vi "process queue.vi"(6 "clear log?":bool, 10 "max log length (1000)":i32=1000, 11 "log queue":refnum<queue>) -> (2 "log items":string[](array[string]), 3 "# of items retrieved":i32)   [LabVIEW 2019, in "WebSocket Echo Server.lvlib"]
uses:
  WebSocket Echo Server.lvlib
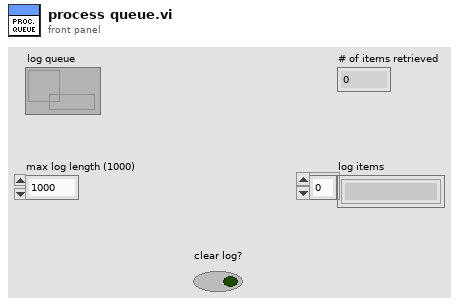
[diagram p1: front panel]
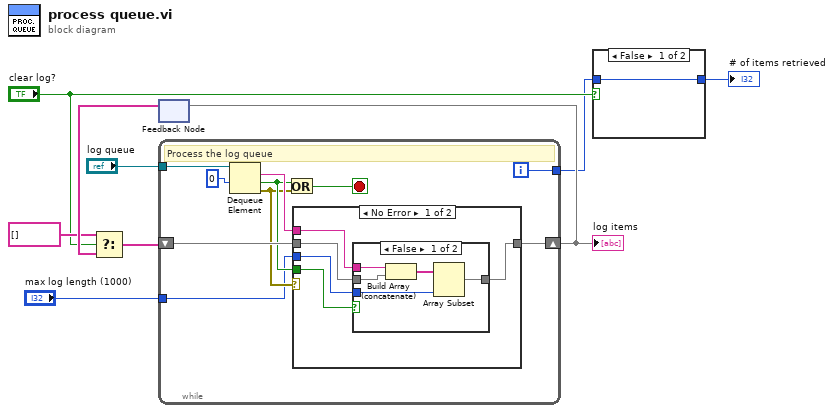
[diagram p0: block diagram]
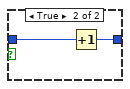
[diagram p2: hidden frame]
diagram:
  n1 = feedback #1() -> (w6:string[])  [unwired: 1 in]
  n2 = Select(t=string[] [], s="clear log?", f=w6) -> (s? t:f=w5:string[])
  n3 = while {
    tunnel: "log queue" -> [w19]
    shift-right: [w16] -> w9
    shift-left: w5 -> [w17]
    tunnel: [w14] -> w2
    tunnel: "max log length (1000)" -> [w10]
    i -> [w14]
    stop <- w11 stop-if-true
    # "Process the log queue"
    n4 = Dequeue Element(queue=w19, timeout in ms (-1)=0) -> (element=w18:string, timed out?=w13:bool, error out=w12:errorcluster)  [unwired: 1 in, 1 out]
    n5 = Or(x=w13, y=w12) -> (x .or. y?=w11:bool)
    n6 = case shown="No Error" w12 {
      tunnel: w13 -> [w23 _]
      tunnel: w18 -> [w24 _]
      tunnel: [w22 w31] -> w16
      tunnel: w17 -> [w21 w31]
      tunnel: w10 -> [w20 _]
      frame No Error {
        n7 = case shown="False" w23 {
          tunnel: w24 -> [w29 _]
          tunnel: [w26 w30] -> w22
          tunnel: w21 -> [w27 w30]
          tunnel: w20 -> [w25 _]
          frame False {
            n8 = Build Array (concatenate)(w29, w27) -> (w28:string[])
            n9 = Array Subset(array=w28, length=w25) -> (w26:string[])  [unwired: 1 in]
          }
          frame True {
          }
        }
      }
      frame Error {
      }
    }
  }
  "log items" <- w9
  n10 = feedback-in #1(w9) -> ()
  n11 = case shown="False" "clear log?" {
    tunnel: w2 -> [w32 w34]
    tunnel: [w32 w33] -> w1
    frame False {
    }
    frame True {
      n12 = Increment(x=w34) -> (x+1=w33:i32)
    }
  }
  "# of items retrieved" <- w1
